vi "流程复合写入.vi"() -> ()   [LabVIEW 2016, in "斯坦道氨氮V2.lvlib"]
uses:
  <vilib>/Utility/miscctls.llb/LVPointTypeDef.ctl
panel:
  in  "流程路径":path=path "data/流程.xml"
  in  "一键写入":bool
  in  "测量模式":enum16{"跨度核查", "水样测量", "零点核查", "标样核查", "加标回收"}(ring)
  out "连接的字符串":string
  in  "参数下拉列表":u16(ring) items=["总磷"=1]
  in  "量程下拉列表":enum16{"低量程", "高量程"}(ring)
  in  "取消":bool
  in  "确认":bool
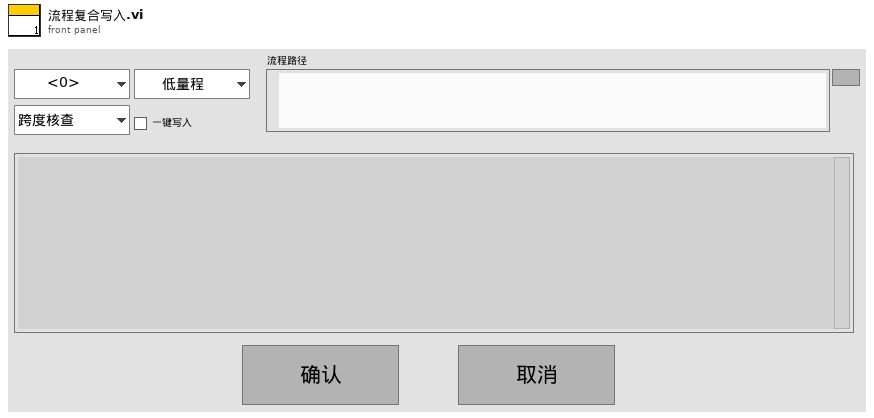
[diagram p1: front panel]
types:
  T1 = typedef "LVPointTypeDef.ctl" = cluster{"Horizontal":i16, "Vertical":i16}
  T2 = typedef "操作日志字段定义.ctl" = cluster{"时间":timestamp, "参数":string, "日志信息":string, "流程参数":string}
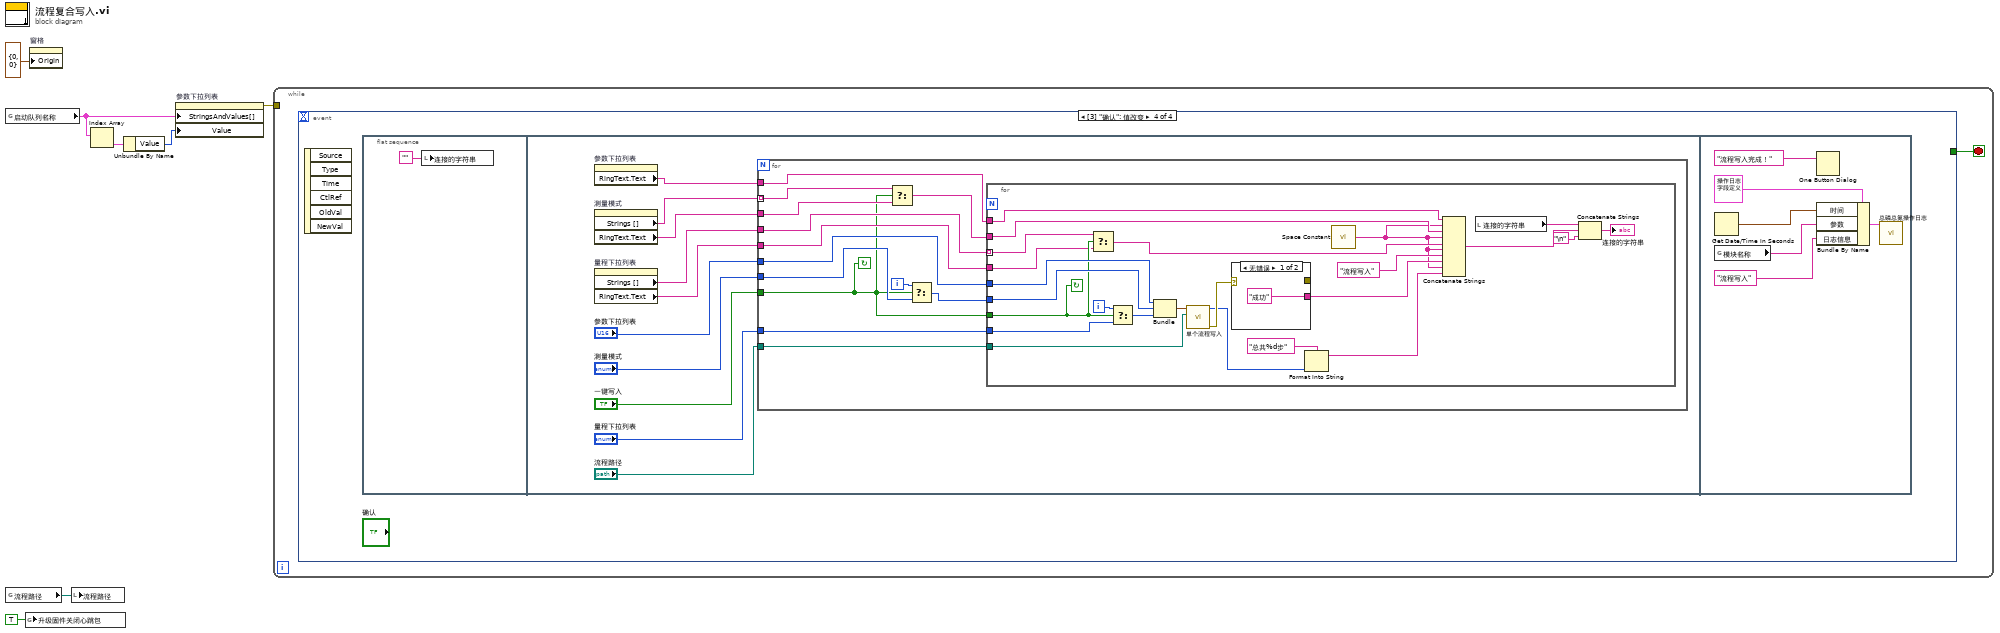
[diagram p0: block diagram]
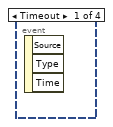
[diagram p2: hidden frame]
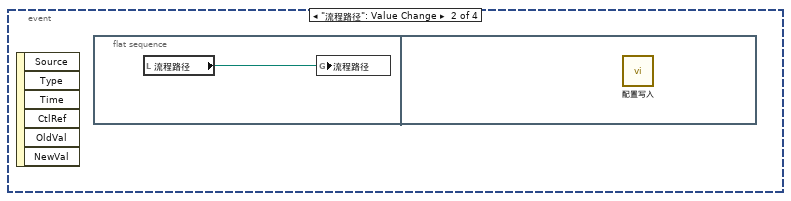
[diagram p3: hidden frame]
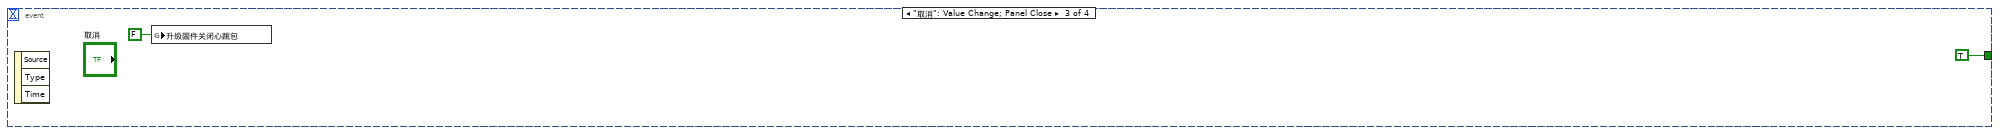
[diagram p4: hidden frame]
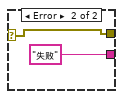
[diagram p5: hidden frame]
diagram:
  n1 = global read "总磷总氮断电保存全局变量.vi" "启动队列名称"() -> (w4:cluster{"String":string, "Value":u16}[])
  n2 = global read "总磷总氮断电保存全局变量.vi" "流程路径"() -> (w5:path)
  n3 = global write "VAR总磷总氮全局变量.vi" "升级固件关闭心跳包"(TRUE ("升级固件关闭心跳包")) -> ()
  n4 = property on="窗格" class="Pane"("Origin"=T1 {"Horizontal"=0, "Vertical"=0} ("原点")) -> ()  [unwired: 2 in, 2 out]
  n5 = local write "流程路径"(w5) -> ()
  n6 = Index Array(array=w4) -> (element=w3:cluster{"String":string, "Value":u16})  [unwired: 1 in]
  n7 = Unbundle By Name(w3) -> ("Value"=w2:u16)
  n8 = property on="参数下拉列表" class="Ring (严格)"("StringsAndValues[]"=w4, "Value"=w2) -> (error out=w6:errorcluster)  [unwired: 2 in, 1 out]
  n9 = while {
    tunnel: w6 -> [_]
    stop <- w8 stop-if-true
    n10 = event shown="[3] \"确认\": 值改变" {
      selector: _ -> [_ _ _ _]
      dyn-events: _ -> [_ _ _ _]
      timeout: _ -> [_ _ _ _]
      tunnel: [_ _ TRUE _] -> w8
      event Timeout {
        n11 = event-data() -> ()  [unwired: 1 in, 3 out]
      }
      event "流程路径": Value Change {
        n12 = event-data() -> ()  [unwired: 1 in, 6 out]
        n13 = flat-sequence {
          frame #0 {
            n14 = local read "流程路径"() -> (w9:path)
            n15 = global write "总磷总氮断电保存全局变量.vi" "流程路径"(w9) -> ()
          }
          frame #1 {
            n16 = call "配置写入.vi"() -> ()  [unwired: 11 in, 1 out]
          }
        }
      }
      event "取消": Value Change; Panel Close {
        n17 = event-data() -> ()  [unwired: 1 in, 3 out]
        n18 = global write "VAR总磷总氮全局变量.vi" "升级固件关闭心跳包"(FALSE ("升级固件关闭心跳包")) -> ()
      }
      event "确认": Value Change {
        n19 = event-data() -> ()  [unwired: 1 in, 6 out]
        n20 = flat-sequence {
          frame #0 {
            n21 = local write "连接的字符串"("") -> ()
          }
          frame #1 {
            n22 = property on="参数下拉列表" class="Ring (严格)"() -> ("RingText.Text"=w16:string)  [unwired: 2 in, 2 out]
            n23 = property on="测量模式" class="Enum (严格)"() -> ("Strings []"=w20:string[], "RingText.Text"=w19:string)  [unwired: 2 in, 2 out]
            n24 = property on="量程下拉列表" class="Enum (严格)"() -> ("Strings []"=w13:string[], "RingText.Text"=w15:string)  [unwired: 2 in, 2 out]
            n25 = for {
              tunnel: "参数下拉列表" -> [w26]
              tunnel: "量程下拉列表" -> [w25]
              tunnel: w20 -> [w33] mode=indexing
              tunnel: w19 -> [w32]
              tunnel: "一键写入" -> [w23]
              tunnel: "测量模式" -> [w34]
              tunnel: w16 -> [w30]
              tunnel: w15 -> [w29]
              tunnel: "流程路径" -> [w28]
              tunnel: w13 -> [w24]
              i -> [w35]
              stop <- w23 continue-if-true
              n26 = Select(t=w33, s=w23, f=w32) -> (s? t:f=w31:string)
              n27 = Select(t=w35, s=w23, f=w34) -> (s? t:f=w27:i32)
              n28 = for {
                tunnel: w31 -> [w53]
                tunnel: w30 -> [w51]
                tunnel: w29 -> [w42]
                tunnel: w28 -> [w50]
                tunnel: w27 -> [w49]
                tunnel: w26 -> [w48]
                tunnel: w25 -> [w47]
                tunnel: w24 -> [w43] mode=indexing
                tunnel: w23 -> [w44]
                i -> [w45]
                stop <- w44 continue-if-true
                n29 = Select(t=w43, s=w44, f=w42) -> (s? t:f=w41:string)
                n30 = Select(t=w45, s=w44, f=w47) -> (s? t:f=w46:i32)
                n31 = Bundle("参数下拉列表"=w48, "测量模式"=w49, "量程下拉列表"=w46) -> (w40:cluster{"参数下拉列表":u16, "测量模式":i32, "量程下拉列表":i32})  [unwired: 1 in]
                n32 = call "单个流程写入.vi"("添加的路径"=w50, "参数簇"=w40) -> ("error out"=w59:errorcluster, "步数"=w37:i32)  [unwired: 8 in]
                n33 = case shown="无错误" w59 {
                  selector: w59 -> [_ w62]
                  tunnel: [_ w62] -> _
                  tunnel: ["成功" "失败"] -> w52
                  frame No Error {
                  }
                  frame Error {
                  }
                }
                n34 = Format Into String(format string="总共%d步" ("格式字符串"), w37) -> (resulting string=w36:string)  [unwired: 2 in, 1 out]
                n35 = call <vilib>:"Space Constant.vi"() -> ("String"=w39:string)
                n36 = Concatenate Strings(w51, w39, w53, w39, w41, w39, "流程写入", w52, w39, w36) -> (w57:string)
                n37 = local read "连接的字符串"() -> (w54:string)
                n38 = Concatenate Strings(w54, w57, "\n") -> (→"连接的字符串":string)
              }
            }
          }
          frame #2 {
            n39 = Get Date/Time In Seconds() -> (seconds since 1Jan1904=w65:timestamp)
            n40 = global read "VAR总磷总氮全局变量.vi" "模块名称"() -> (w64:string)
            n41 = One Button Dialog(message="流程写入完成！" ("消息")) -> ()  [unwired: 1 in, 1 out]
            n42 = Bundle By Name(cluster=T2 {"时间"=timestamp(0 s since 1904-01-01), "参数"="", "日志信息"="", "流程参数"=""} ("data in"), "时间"=w65, "参数"=w64, "日志信息"="流程写入") -> (w66:T2)
            n43 = call "总磷总氮操作日志.vi"("data in"=w66) -> ()  [unwired: 10 in, 1 out]
          }
        }
      }
    }
  }
